vi "Get ResultS of the Proccess from URL link.vi"(8 "error in":errorcluster, 9 "Proccess":string[](array[string]), 10 "Serial number":string, 11 "Models":string) -> (0 "error out":errorcluster, 3 "Results of the Proccess":string[](array[string]))   [LabVIEW 2025, in "MES Interlcok.lvlib"]
uses:
  MES Interlcok.lvlib
  <vilib>/httpClient/LabVIEWHTTPClient.lvlib
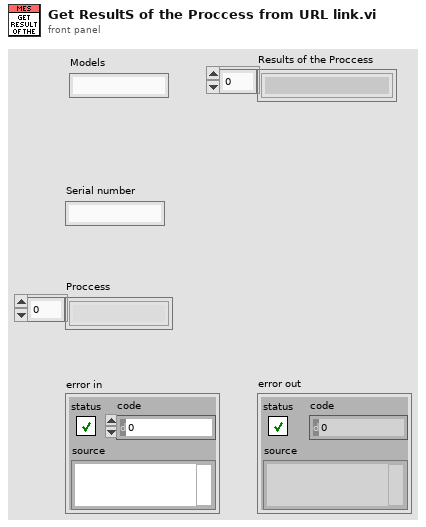
[diagram p1: front panel]
types:
  T1 = typedef "LabVIEWHTTPClient.lvlib/ClientHandle.ctl" = refnum<k1>
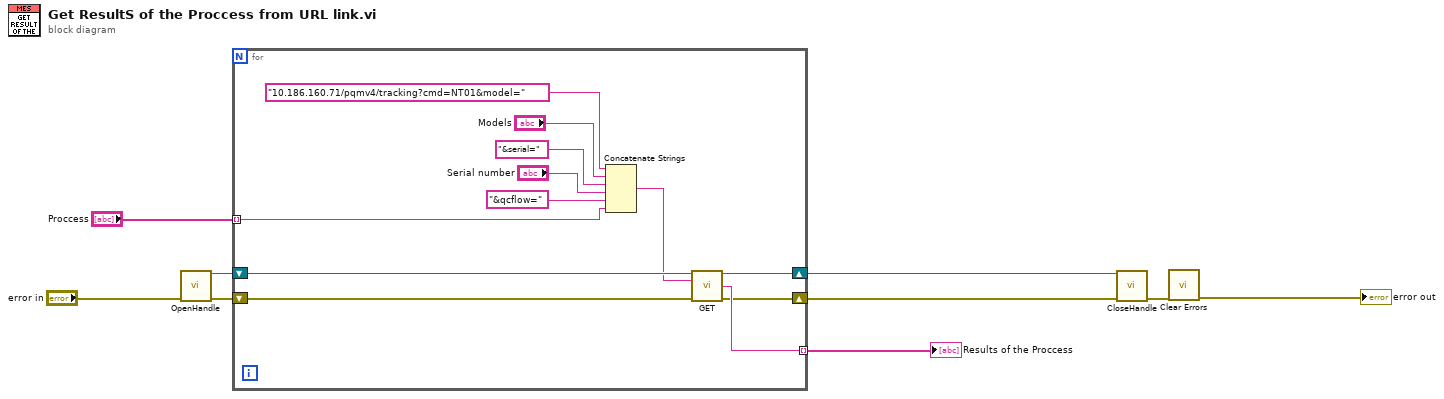
[diagram p0: block diagram]
diagram:
  n1 = call <vilib>:"OpenHandle.vi"("error in (no error)"="error in") -> ("client handle out"=w9:T1, "error out"=w8:errorcluster)  [unwired: 13 in]
  n2 = for {
    tunnel: [w19] -> w7 mode=indexing
    shift-right: [w18] -> w6
    shift-left: w9 -> [w21]
    shift-right: [w17] -> w5
    shift-left: w8 -> [w20]
    tunnel: "Proccess" -> [w10] mode=indexing
    n3 = Concatenate Strings("10.186.160.71/pqmv4/tracking?cmd=NT01&model=", "Models", "&serial=", "Serial number", "&qcflow=", w10) -> (w12:string)
    n4 = call <vilib>:"GET.vi"("client handle"=w21, "url"=w12, "error in (no error)"=w20) -> ("client handle out"=w18:T1, "body"=w19:string, "error out"=w17:errorcluster)  [unwired: 9 in, 1 out]
  }
  "Results of the Proccess" <- w7
  n5 = call <vilib>:"CloseHandle.vi"("client handle"=w6, "error in (no error)"=w5) -> ("error out"=w3:errorcluster)  [unwired: 13 in]
  n6 = call <vilib>:"Clear Errors.vi"("error in (no error)"=w3) -> ("error out"=→"error out":errorcluster)  [unwired: 5 in, 1 out]
